vi "GitLog.vi"(6 "GetCurrentTag(T)":bool, 8 "error in (no error)":errorcluster, 11 "Directory (leave empty for relative)":path) -> (0 "error out":errorcluster, 3 "directory out":path, 5 "git log":string, 7 "tag":string)   [LabVIEW 2018]
panel:
  out "comp":string
  out "standard error":string
  out "commit":string
  out "standard output":string
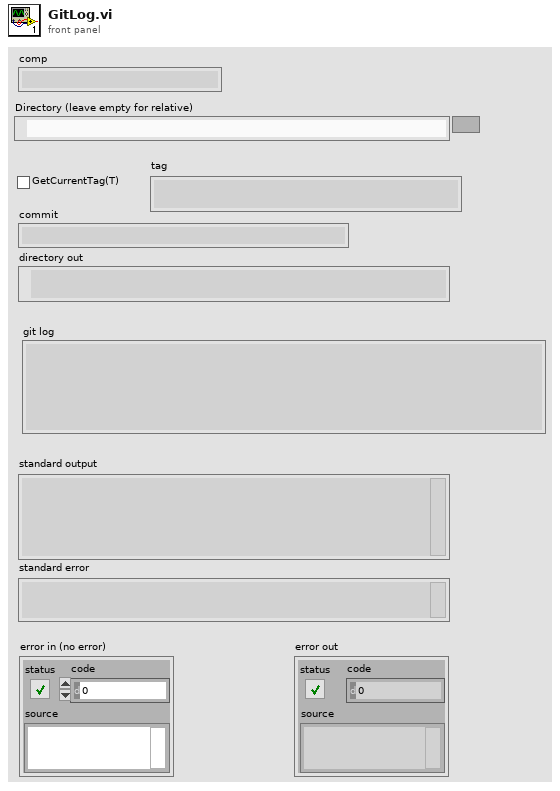
[diagram p1: front panel]
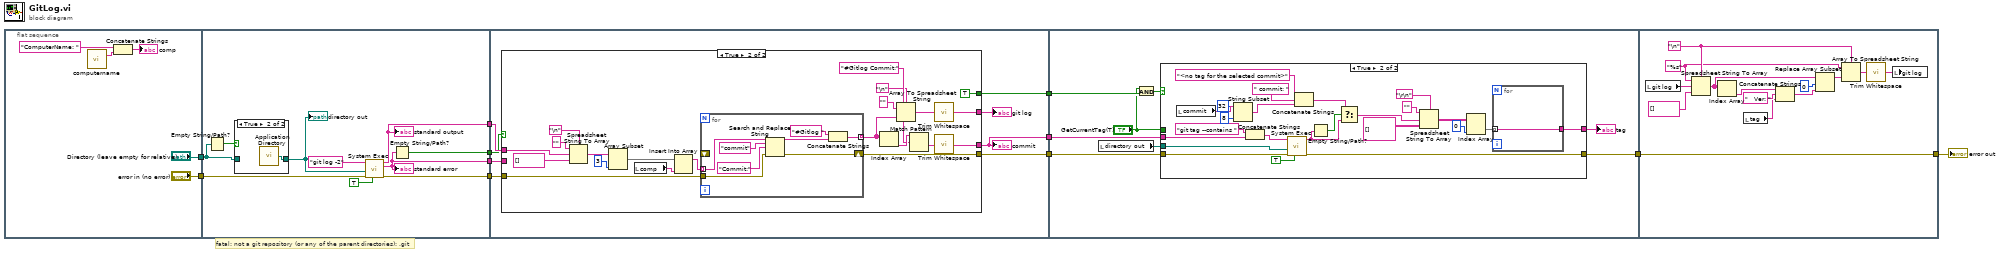
[diagram p0: block diagram]
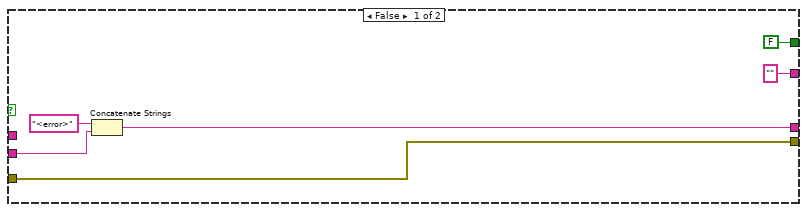
[diagram p3: hidden frame]
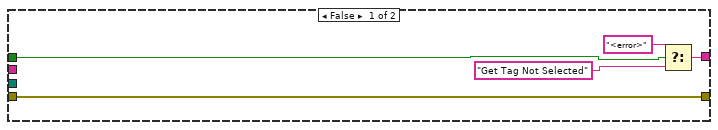
[diagram p4: hidden frame]
diagram:
  # "fatal: not a git repository (or any of the parent directories): .git"
  n1 = flat-sequence {
    tunnel: ["error in (no error)"] -> w11
    tunnel: ["Directory (leave empty for relative)"] -> w10
    tunnel: w11 -> [w23]
    tunnel: w10 -> [w21]
    tunnel: [w25] -> w9
    tunnel: [w22] -> w8
    tunnel: [w18] -> w4
    tunnel: [w17] -> w3
    tunnel: w9 -> [w35]
    tunnel: w8 -> [w32]
    tunnel: [w34] -> w7
    tunnel: [w33] -> w5
    tunnel: w4 -> [w31]
    tunnel: w3 -> [w30]
    tunnel: [w29] -> w2
    tunnel: w7 -> [w79]
    tunnel: w5 -> [w76]
    tunnel: w2 -> [w74]
    tunnel: [w77] -> w1
    tunnel: [w123] -> w6
    tunnel: w1 -> [w123]
    frame #0 {
      n2 = call "computername.vi"() -> ("String/Binary data"=w13:string)  [unwired: 4 in, 1 out]
      n3 = Concatenate Strings("ComputerName: " ("string"), w13) -> (→"comp":string)
    }
    frame #1 {
      n4 = Empty String/Path?(string/path=w21) -> (empty?=w20:bool)
      n5 = case shown="True" w20 {
        tunnel: [w27 w28] -> w19
        tunnel: w21 -> [w27 _]
        frame False {
        }
        frame True {
          n6 = call <vilib>:"Application Directory.vi"() -> ("Application Directory"=w28:path)
        }
      }
      "directory out" <- w19
      n7 = call <vilib>:"System Exec.vi"("run minimized? (F)"=TRUE, "error in (no error)"=w23, "working directory"=w19, "command line"="git log -2") -> ("error out"=w22:errorcluster, "standard error"=w17:string, "standard output"=w25:string)  [unwired: 4 in, 1 out]
      "standard output" <- w25
      "standard error" <- w17
      n8 = Empty String/Path?(string/path=w17) -> (empty?=w18:bool)
    }
    frame #2 {
      n9 = case shown="True" w31 {
        tunnel: ["" ("spreadsheet string") w43] -> w36
        tunnel: w35 -> [_ w49]
        tunnel: [w39 w47] -> w34
        tunnel: [w42 w46] -> w33
        tunnel: w32 -> [w42 w45]
        tunnel: w30 -> [w38 _]
        tunnel: [FALSE ("y") TRUE ("y")] -> w29
        frame False {
          n10 = Concatenate Strings("<error>" ("trimmed string"), w38) -> (w39:string)
        }
        frame True {
          n11 = Spreadsheet String To Array(delimiter (Tab)="\n", format string="", spreadsheet string=w49, array type (2D Dbl)=string[] []) -> (array=w56:string[])
          n12 = Array Subset(array=w56, length=3) -> (w57:string[])  [unwired: 1 in]
          n13 = local read "comp"() -> (w63:string)
          n14 = Insert Into Array(array=w57, new element=w63) -> (w58:string[])  [unwired: 1 in]
          n15 = for {
            tunnel: w58 -> [w69] mode=indexing
            tunnel: [w70] -> w60 mode=indexing
            shift-right: [w65] -> w46
            shift-left: _ -> [_]
            tunnel: w45 -> [w64]
            n16 = Search and Replace String(input string=w69, search string="commit", replace string="Commit:" ("replace string (\"\")"), error in=w64) -> (result string=w67:string, error out=w65:errorcluster)  [unwired: 4 in, 2 out]
            n17 = Concatenate Strings("#Gitlog " ("string"), w67) -> (w70:string)
          }
          n18 = Index Array(array=w60) -> (element=w61:string)  [unwired: 1 in]
          n19 = Array To Spreadsheet String(delimiter (Tab)="\n", array=w60, 3:"" ("format string")) -> (spreadsheet string=w59:string)
          n20 = Match Pattern(string=w61, regular expression="#Gitlog Commit:") -> (after substring=w62:string)  [unwired: 1 in, 3 out]
          n21 = call <vilib>:"Trim Whitespace.vi"("string"=w59) -> ("trimmed string"=w43:string)  [unwired: 1 in]
          n22 = call <vilib>:"Trim Whitespace.vi"("string"=w62) -> ("trimmed string"=w47:string)  [unwired: 1 in]
        }
      }
      "git log" <- w36
      "commit" <- w34
    }
    frame #3 {
      n23 = local read "directory out"() -> (w78:path)
      n24 = And(x="GetCurrentTag(T)", y=w74) -> (x .and. y?=w75:bool)
      n25 = case shown="True" w75 {
        tunnel: w79 -> [_ w106]
        tunnel: w78 -> [_ w104]
        tunnel: [w83 w97] -> w72
        tunnel: [w84 w100] -> w77
        tunnel: w76 -> [w84 w99]
        tunnel: "GetCurrentTag(T)" -> [w82 _]
        frame False {
          n26 = Select(t="<error>" ("standard output"), s=w82, f="Get Tag Not Selected") -> (s? t:f=w83:string)
        }
        frame True {
          n27 = local read "commit"() -> (w90:string)
          n28 = String Subset(string=w90, offset (0)=32, length (rest)=8 ("length (rest)")) -> (substring=w87:string)
          n29 = Concatenate Strings("git tag --contains " ("command line"), w106) -> (w107:string)
          n30 = call <vilib>:"System Exec.vi"("run minimized? (F)"=TRUE, "error in (no error)"=w99, "working directory"=w104, "command line"=w107) -> ("error out"=w100:errorcluster, "standard output"=w102:string)  [unwired: 4 in, 2 out]
          n31 = Concatenate Strings("<no tag for the selected commit>" ("t"), " commit: " ("t"), w87) -> (w88:string)
          n32 = Empty String/Path?(string/path=w102) -> (empty?=w103:bool)
          n33 = Select(t=w88, s=w103, f=w102) -> (s? t:f=w98:string)
          n34 = Spreadsheet String To Array(delimiter (Tab)="\r\n", format string="", spreadsheet string=w98, array type (2D Dbl)=string[][] []) -> (array=w93:string[][])
          n35 = Index Array(array=w93, index (col)=0 ("disabled index (col)")) -> (element=w94:string[])  [unwired: 1 in]
          n36 = for {
            tunnel: w94 -> [w109] mode=indexing
            tunnel: [w109] -> w97
          }
        }
      }
      "tag" <- w72
    }
    frame #4 {
      w113 = "\n"
      w112 = "%s" ("format string")
      n37 = local read "git log"() -> (w122:string)
      n38 = Spreadsheet String To Array(delimiter (Tab)=w113, format string=w112, spreadsheet string=w122, array type (2D Dbl)=string[] []) -> (array=w117:string[])
      n39 = Index Array(array=w117) -> (element=w120:string)  [unwired: 1 in]
      n40 = local read "tag"() -> (w118:string)
      n41 = Concatenate Strings(w120, "   Ver: " ("string"), w118) -> (w116:string)
      n42 = Replace Array Subset(array=w117, new element=w116, index=0) -> (w114:string[])
      n43 = Array To Spreadsheet String(delimiter (Tab)=w113, array=w114, 3:w112) -> (spreadsheet string=w110:string)
      n44 = call <vilib>:"Trim Whitespace.vi"("string"=w110) -> ("trimmed string"=w111:string)  [unwired: 1 in]
      n45 = local write "git log"(w111) -> ()
    }
  }
  "error out" <- w6
